vi "Check.vi"(4 "error in (no error)":errorcluster, 5 "Type":string, 6 "Wafer ID":string, 7 "LotData in":refnum<class "LotData.lvclass">) -> (0 "error out":errorcluster, 1 "Tested?":bool, 2 "Exists?":bool, 3 "LotData out":refnum<class "LotData.lvclass">)   [LabVIEW 2012, in "LotData.lvclass"]
uses:
  Classes/LotData.lvclass
  Classes/LotData.lvclass/LotData.ctl
  <vilib>/addons/database/Connection.llb/DB Tools Open Connec (Path).vi
  <vilib>/addons/database/Connection.llb/Conn Execute.vi
  <vilib>/addons/database/Recordset.llb/Rec Fetch Recordset Data (R).vi
  <vilib>/addons/database/Recordset.llb/Rec Destroy - Connection.vi
  <vilib>/addons/database/NI_Database_API.lvlib
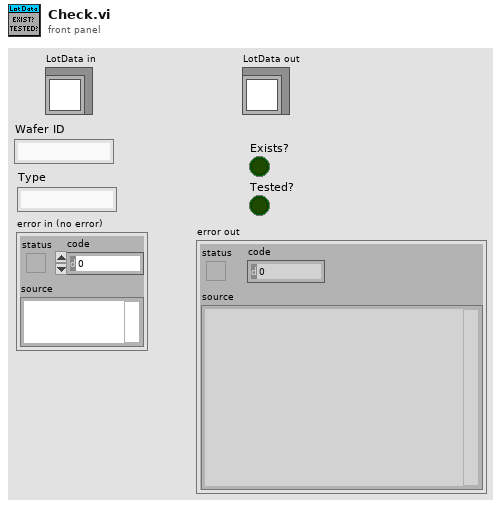
[diagram p1: front panel]
types:
  T1 = typedef "NI_Database_API.lvlib/Conn ObjectReference.ctl" = refnum<k1>
  T2 = typedef "NI_Database_API.lvlib/Rec ObjectReference.ctl" = refnum<k1>
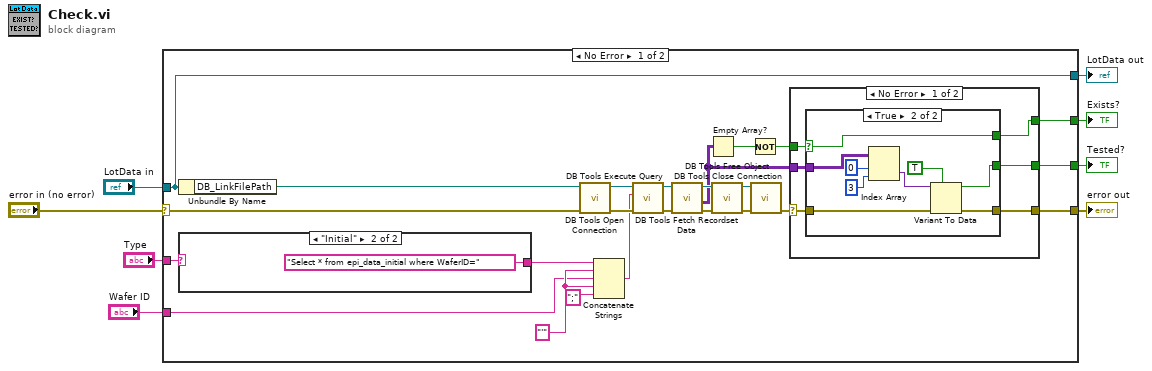
[diagram p0: block diagram]
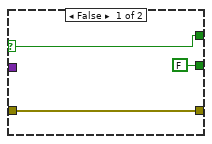
[diagram p2: hidden frame]
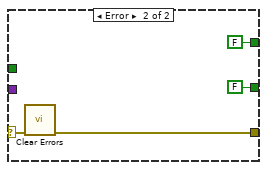
[diagram p3: hidden frame]
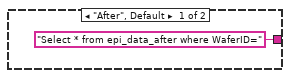
[diagram p4: hidden frame]
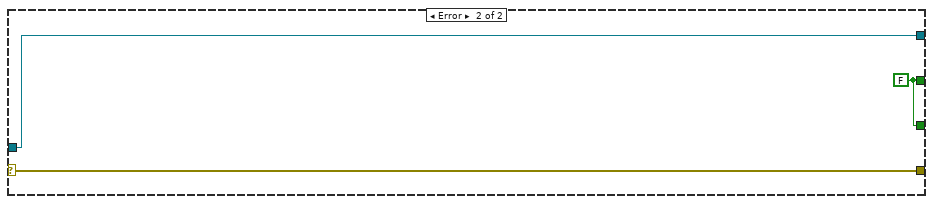
[diagram p5: hidden frame]
diagram:
  n1 = case shown="No Error" "error in (no error)" {
    selector: "error in (no error)" -> [w15 w59]
    tunnel: [w13 w59] -> w7
    tunnel: [w9 w58] -> w5
    tunnel: "LotData in" -> [w9 w58]
    tunnel: [w12 w57] -> w4
    tunnel: [w14 w57] -> w3
    tunnel: "Wafer ID" -> [w11 _]
    tunnel: "Type" -> [w17 _]
    frame No Error {
      w23 = "'" ("string")
      n2 = Unbundle By Name(w9) -> ("DB_LinkFilePath"=w10:path)
      n3 = case shown="\"Initial\"" w17 {
        tunnel: ["Select * from epi_data_after where WaferID=" ("string") "Select * from epi_data_initial where WaferID=" ("string")] -> w16
        frame "After", Default {
        }
        frame "Initial" {
        }
      }
      n4 = call-poly <vilib>:"DB Tools Open Connection.vi"("error in (no error)"=w15, "connection information"=w10) -> ("error out"=w31:errorcluster, "connection reference"=w32:T1)  [unwired: 6 in]
      n5 = Concatenate Strings(w16, w23, w11, w23, ";" ("string")) -> (w24:string)
      n6 = call-poly <vilib>:"DB Tools Execute Query.vi"("error in (no error)"=w31, "SQL query"=w24, "connection reference"=w32) -> ("error out"=w27:errorcluster, "recordset reference"=w28:T2)  [unwired: 5 in]
      n7 = call-poly <vilib>:"DB Tools Fetch Recordset Data.vi"("error in (no error)"=w27, "recordset reference"=w28) -> ("error out"=w25:errorcluster, "recordset data"=w18:variant[][], "recordset reference out"=w26:T2)  [unwired: 3 in]
      n8 = Empty Array?(array=w18) -> (empty?=w21:bool)
      n9 = call-poly <vilib>:"DB Tools Free Object.vi"("error in (no error)"=w25, "recordset reference"=w26) -> ("error out"=w29:errorcluster, "connection reference"=w30:T1)  [unwired: 8 in]
      n10 = Not(x=w21) -> (.not. x?=w19:bool)
      n11 = call <vilib>:"DB Tools Close Connection.vi"("error in (no error)"=w29, "connection reference"=w30) -> ("error out"=w20:errorcluster)  [unwired: 5 in]
      n12 = case shown="No Error" w20 {
        selector: w20 -> [w35 w54]
        tunnel: w19 -> [w38 _]
        tunnel: [w36 w53] -> w13
        tunnel: w18 -> [w37 _]
        tunnel: [w34 FALSE] -> w14
        tunnel: [w33 FALSE] -> w12
        frame No Error {
          n13 = case shown="True" w38 {
            selector: w38 -> [w39 w42]
            tunnel: w37 -> [_ w50]
            tunnel: [w41 w46] -> w36
            tunnel: w35 -> [w41 w45]
            tunnel: [FALSE w43] -> w34
            tunnel: [w39 w42] -> w33
            frame False {
            }
            frame True {
              n14 = Index Array(array=w50, index (row)=0, index (col)=3 ("disabled index (col)")) -> (element=w47:variant)
              n15 = Variant To Data(error in=w45, type=TRUE, Variant=w47) -> (data=w43:bool, error out=w46:errorcluster)
            }
          }
        }
        frame Error {
          n16 = call <vilib>:"Clear Errors.vi"("error in (no error)"=w54) -> ("error out"=w53:errorcluster)  [unwired: 6 in]
        }
      }
    }
    frame Error {
      w57 = FALSE
    }
  }
  "error out" <- w7
  "LotData out" <- w5
  "Exists?" <- w4
  "Tested?" <- w3
